vi "Configure Frequency.vi"(7 "Mode":enum16{"Center Span", "Start Stop"}(ring), 8 "error in (no error)":errorcluster, 9 "Span/Stop Frequency":dbl, 10 "Center/Start Frequency":dbl, 11 "VNA-Ag87xx in":refnum<class "VNA-Ag87xx.lvclass">) -> (0 "error out":errorcluster, 3 "VNA-Ag87xx out":refnum<class "VNA-Ag87xx.lvclass">)   [LabVIEW 2020, in "VNA-Ag87xx.lvclass"]
doc: "Configures the frequency range for the sweep.\nThe default mode is Center Span."
uses:
  VNA-Ag87xx.lvclass
  C:/Sandbox/RF Bench/Source Code/WiSpry Test Framework/Instruments/Instrument.lvclass
  C:/Sandbox/RF Bench/Source Code/WiSpry Test Framework/Instruments/Vector Network Analyzer/Vector Network Analyzer.lvclass
  Instrument.lvclass/Instrument.ctl
  Vector Network Analyzer.lvclass/Vector Network Analyzer.ctl
  Instrument.lvclass
  Vector Network Analyzer.lvclass
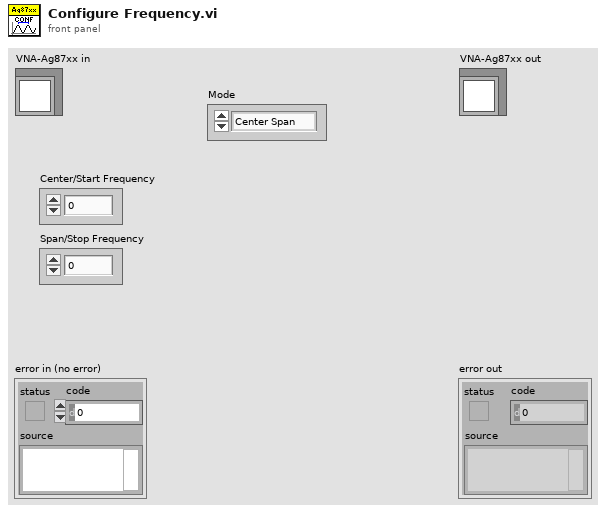
[diagram p1: front panel]
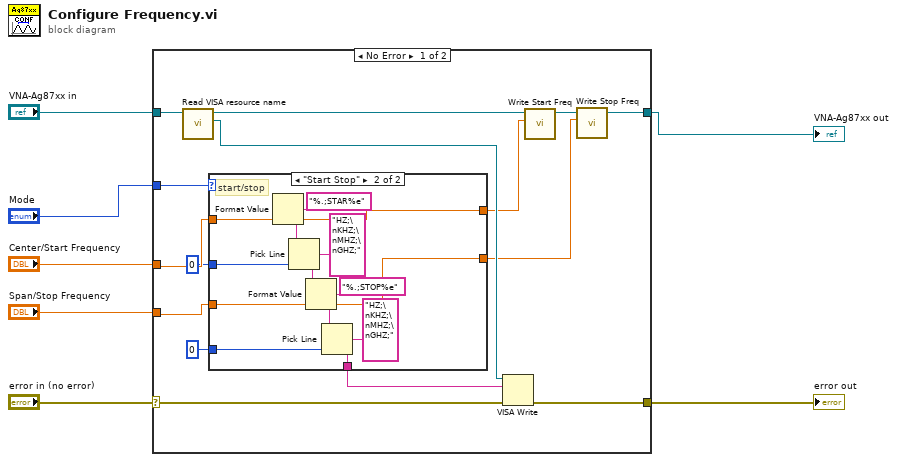
[diagram p0: block diagram]
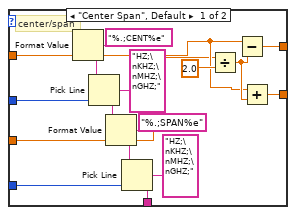
[diagram p2: hidden frame]
diagram:
  n1 = case shown="No Error" "error in (no error)" {
    selector: "error in (no error)" -> [w20 w51]
    tunnel: [w18 w52] -> w5
    tunnel: "VNA-Ag87xx in" -> [w22 w52]
    tunnel: [w21 w51] -> w6
    tunnel: "Span/Stop Frequency" -> [w14 _]
    tunnel: "Center/Start Frequency" -> [w13 _]
    tunnel: "Mode" -> [w10 _]
    frame No Error {
      n2 = call "Read VISA resource name.vi"("Instrument in"=w22) -> ("VISA resource name"=w16:refnum<visa-resource-name>, "Instrument out"=w19:refnum<class "VNA-Ag87xx.lvclass">)  [unwired: 9 in]
      n3 = case shown="\"Start Stop\"" w10 {
        tunnel: w13 -> [w26 w40]
        tunnel: u16 0 ("start/center units (1 : Hz/dBm)") -> [w35 w47]
        tunnel: w14 -> [w25 w39]
        tunnel: u16 0 ("stop/span units (0 : Hz/dBm)") -> [w30 w42]
        tunnel: [w29 w41] -> w15
        tunnel: [w24 w40] -> w9
        tunnel: [w23 w39] -> w8
        frame "Center Span", Default {
          # "center/span"
          n4 = Format Value(format string="%.;CENT%e", value (0)=w26) -> (output string=w37:string)  [unwired: 1 in]
          n5 = Pick Line(string ("")=w37, multi-line string="HZ;\nKHZ;\nMHZ;\nGHZ;", line index=w35) -> (output string=w31:string)
          n6 = Format Value(string ("")=w31, format string="%.;SPAN%e", value (0)=w25) -> (output string=w33:string)
          n7 = Pick Line(string ("")=w33, multi-line string="HZ;\nKHZ;\nMHZ;\nGHZ;", line index=w30) -> (output string=w29:string)
          n8 = Divide(x=w25, y=2.0) -> (x/y=w27:dbl)
          n9 = Subtract(x=w26, y=w27) -> (x-y=w24:dbl)
          n10 = Add(x=w26, y=w27) -> (x+y=w23:dbl)
        }
        frame "Start Stop" {
          # "start/stop"
          n11 = Format Value(format string="%.;STAR%e", value (0)=w40) -> (output string=w49:string)  [unwired: 1 in]
          n12 = Pick Line(string ("")=w49, multi-line string="HZ;\nKHZ;\nMHZ;\nGHZ;", line index=w47) -> (output string=w43:string)
          n13 = Format Value(string ("")=w43, format string="%.;STOP%e", value (0)=w39) -> (output string=w45:string)
          n14 = Pick Line(string ("")=w45, multi-line string="HZ;\nKHZ;\nMHZ;\nGHZ;", line index=w42) -> (output string=w41:string)
        }
      }
      n15 = VISA Write(VISA resource name=w16, write buffer=w15, error in (no error)=w20) -> (error out=w21:errorcluster)  [unwired: 2 out]
      n16 = call "Write Start Freq.vi"("Start Freq"=w9, "Vector Network Analyzer in"=w19) -> ("Vector Network Analyzer out"=w17:refnum<class "VNA-Ag87xx.lvclass">)  [unwired: 9 in]
      n17 = call "Write Stop Freq.vi"("Stop Freq"=w8, "Vector Network Analyzer in"=w17) -> ("Vector Network Analyzer out"=w18:refnum<class "VNA-Ag87xx.lvclass">)  [unwired: 9 in]
    }
    frame Error {
    }
  }
  "error out" <- w6
  "VNA-Ag87xx out" <- w5
